vi "LoopVI-V3.vi"() -> ()   [LabVIEW 2013]
uses:
  <vilib>/Utility/file.llb/Read From Spreadsheet File (DBL).vi
panel:
  out "x*y":dbl
  out "Numeric":dbl format="%#_2f"
  in  "file path (dialog if empty)":path
  in  "Load":bool caption="measurement file\n\n         ??. txt"
  out "free gas model":cluster{"Y":dbl[], "Y":dbl[]}[](graph)
  in  "Fermi angle\n   (mrad)":dbl=7.0
  in  "stop 2":bool
  out "core electrons":cluster{"Y":dbl[], "Y":dbl[]}[](graph)
  in  "core width\n   (mrad)":dbl=5.0
  in  "fraction core\nannihilations":dbl=0.2 min=0.0 max=1.0 step=1e-05
  out "ZICHT  functie":cluster{"Y":dbl[], "Y":dbl[]}[](graph)
  in  "spleetbreedte\n      (mm)":dbl=1.0 min=0.1 max=5.0
  in  "collimator afstand\n       (mm)":dbl=500.0 min=100.0 max=1000.0
  in  "stop 4":bool
  out "XY Graph 4":cluster{ext[], "Array out":ext[]}[](graph)
  in  "alignment correction":dbl min=-10.0 max=10.0 step=0.0001
  in  "background \n coincidence counts":dbl min=0.0 max=100.0
  out "Fermi energy (eV)":dbl format="%#_3g"
  in  "22Na source radius (mm)":dbl=0.1 min=1e-05 max=3.0
  out "?":dbl format="%#_3g"
  in  "1d - Acar":bool caption="2d - Acar or DB"
  out "2d - Acar 2":bool
  out "2d - Acar 3":bool
  out "2d - Acar 4":bool
  out "XY Graph 5":cluster{ext[], "Array out":ext[]}[](graph)
  out "output cluster 2":cluster{ext[], ext[]}
  out "Sum of squared residuals":dbl
  in  "sigma (mrad) 2":dbl
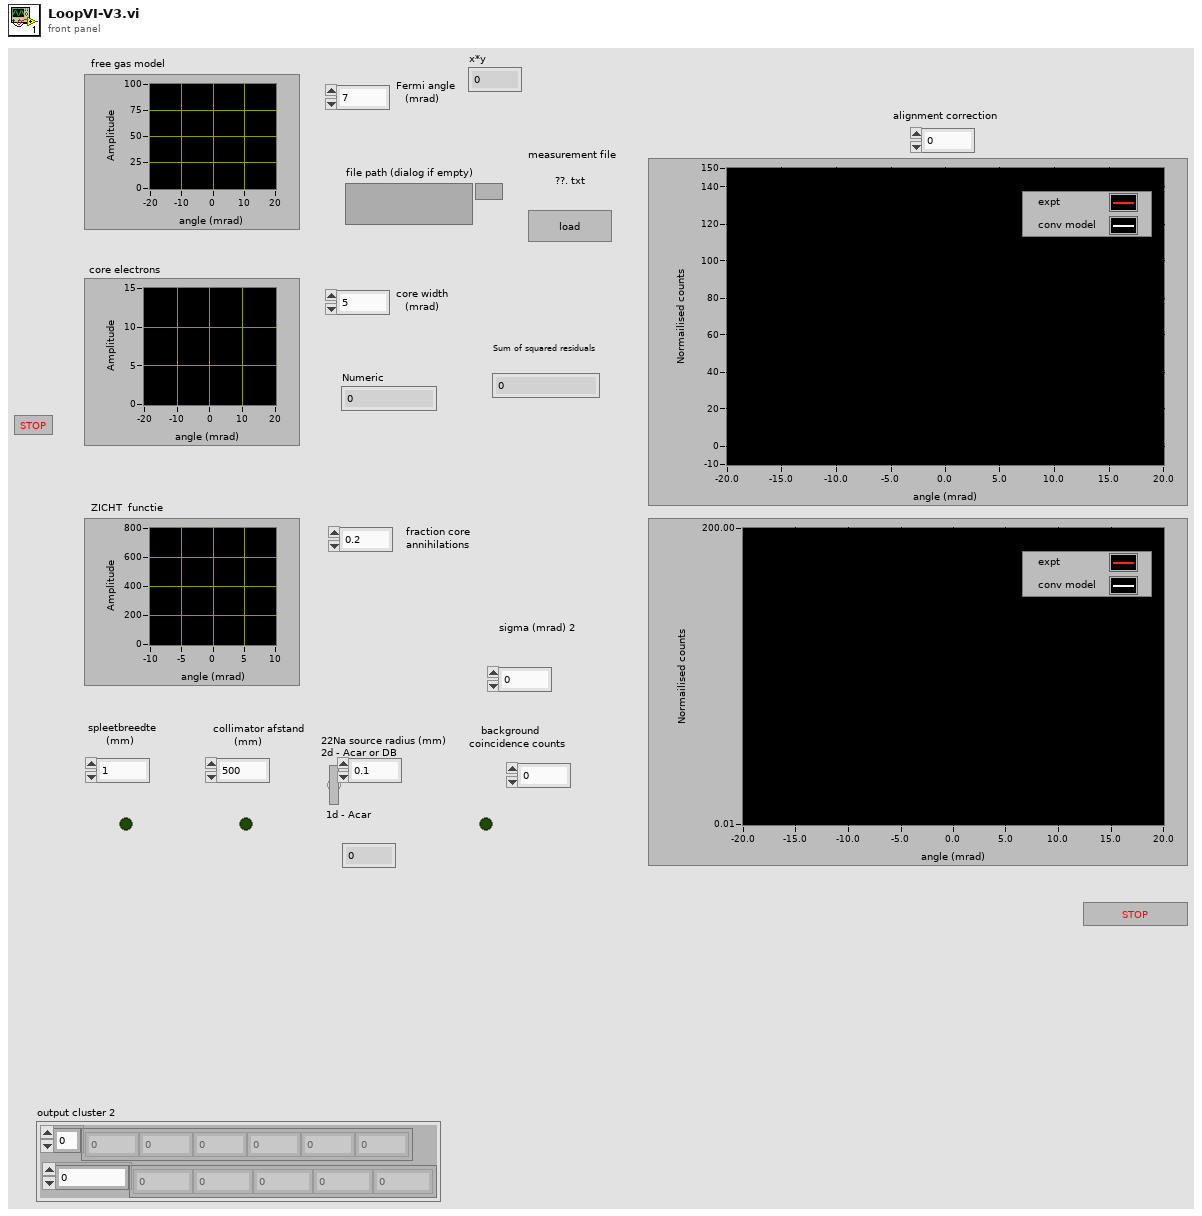
[diagram p1: front panel]
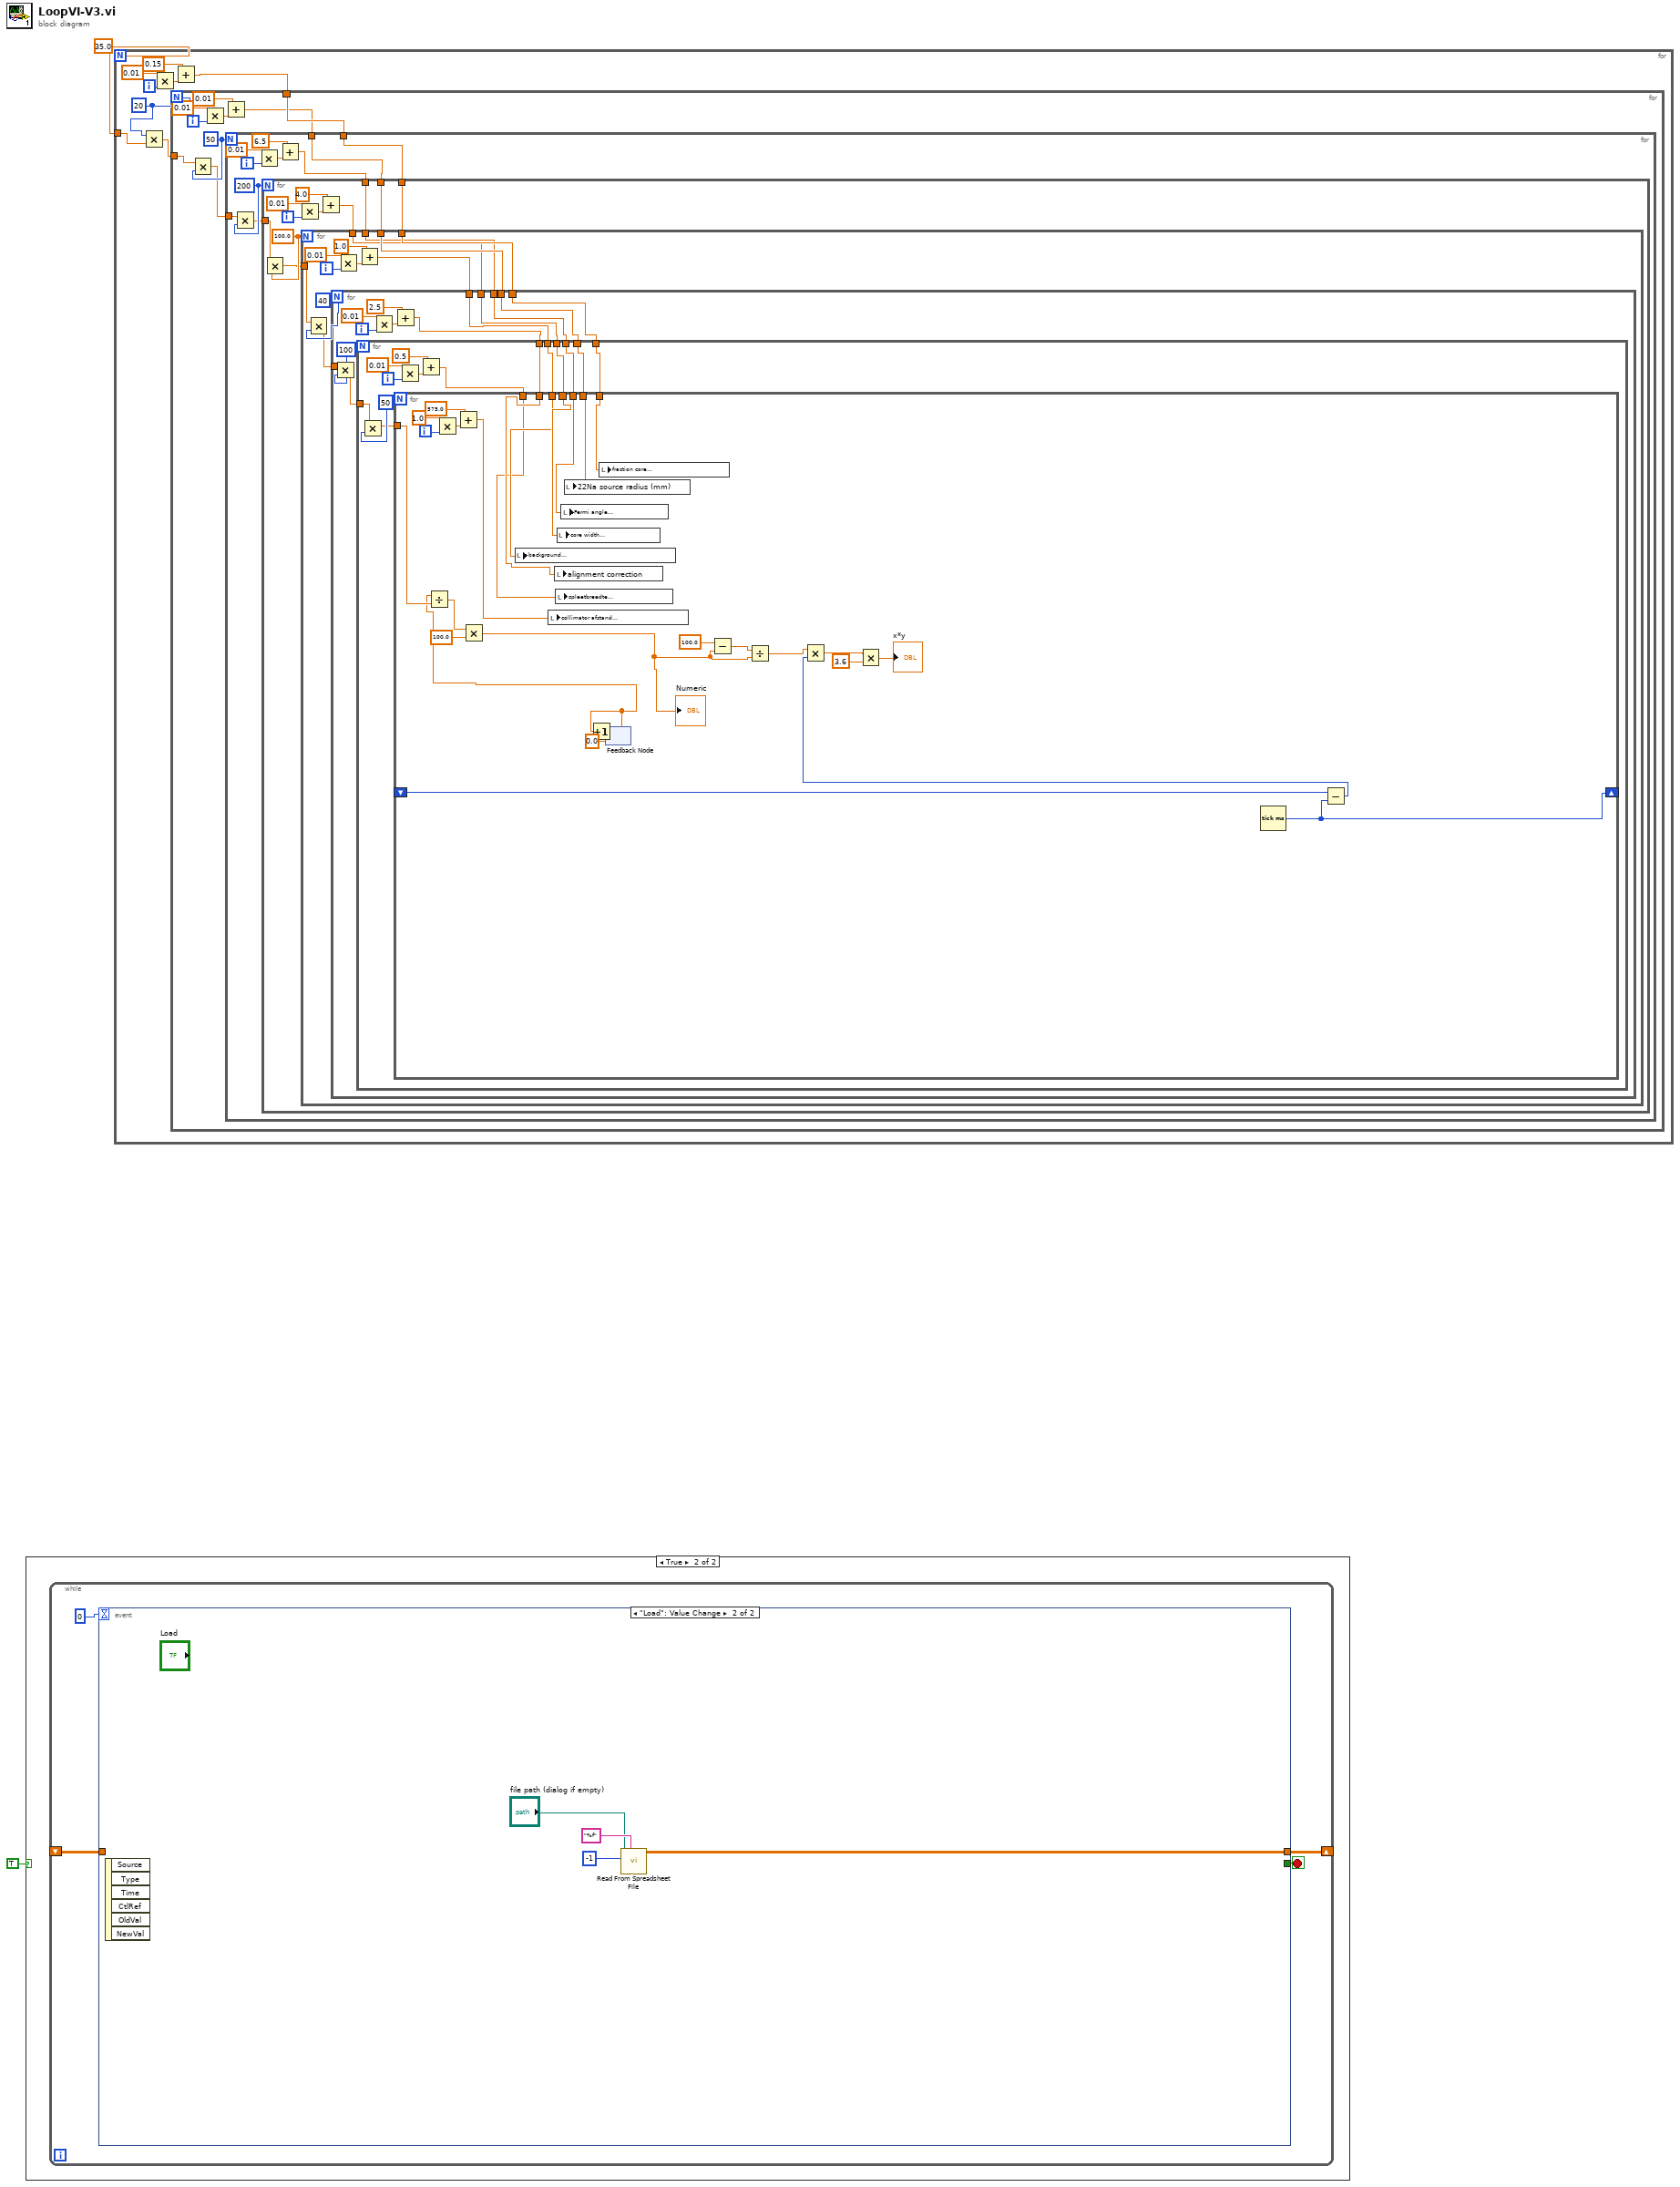
[diagram p0: block diagram]
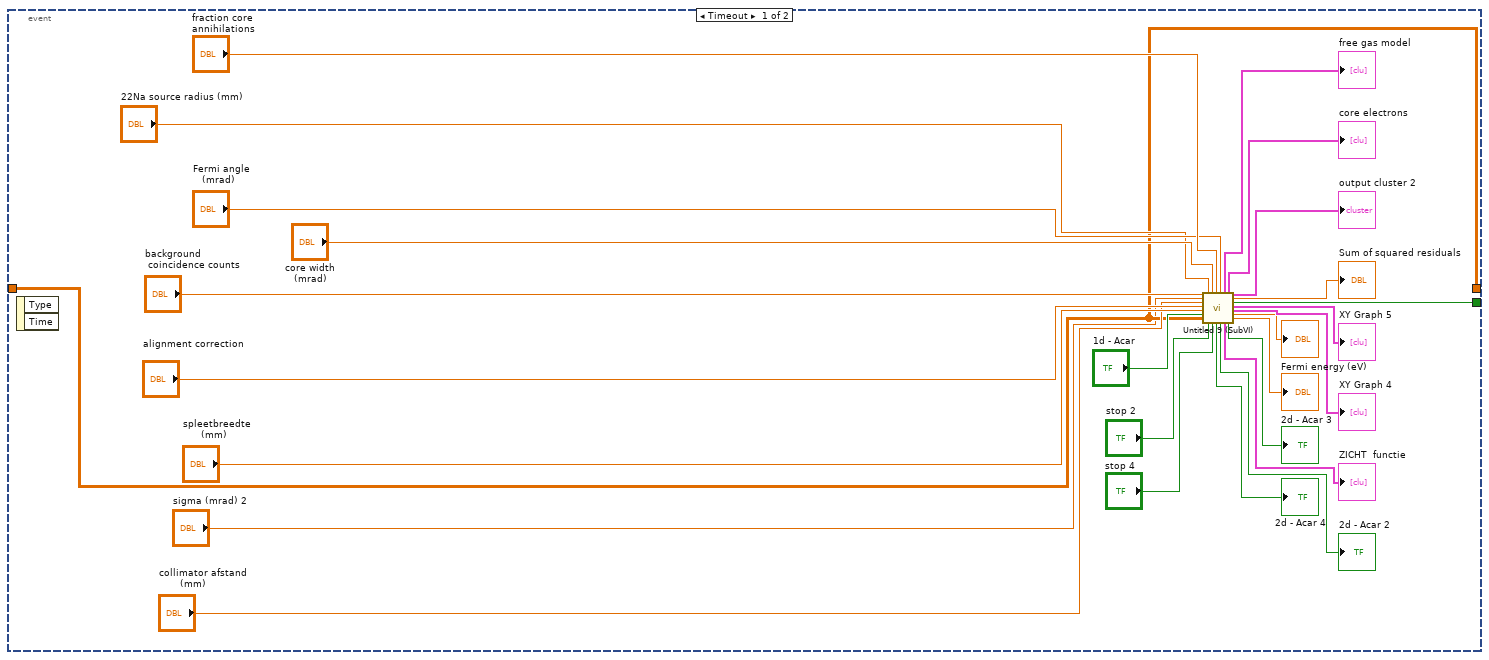
[diagram p3: hidden frame]
diagram:
  w1 = 35.0
  n1 = case shown="True" TRUE {
    frame False {
    }
    frame True {
      n2 = while {
        shift-right: [w4] -> _
        shift-left: _ -> [w3]
        stop <- w6 stop-if-true
        n3 = event shown="[1] \"Load\": Value Change" {
          selector: _ -> [_ _]
          dyn-events: _ -> [_ _]
          timeout: 0 -> [_ _]
          tunnel: [w32 _] -> w6
          tunnel: [w22 w35] -> w4
          tunnel: w3 -> [w22 _]
          event Timeout {
            n4 = event-data() -> ()  [unwired: 1 in, 2 out]
            n5 = call "Untitled 9 (SubVI).vi"("background \n coincidence counts"="background \n coincidence counts", "sigma (mrad) in"="sigma (mrad) 2", "collimator afstand\n       (mm)"="collimator afstand\n       (mm)", "alignment correction"="alignment correction", "spleetbreedte\n      (mm)"="spleetbreedte\n      (mm)", "1d - Acar"="1d - Acar", "all rows"=w22, "22Na source radius (mm)"="22Na source radius (mm)", "stop in"="stop 2", "core width\n   (mrad)"="core width\n   (mrad)", "stop 4"="stop 4", "fraction core\nannihilations"="fraction core\nannihilations", "Fermi angle\n   (mrad)"="Fermi angle\n   (mrad)") -> ("2d - Acar 4"=→"2d - Acar 4":bool, "2d - Acar 2"=→"2d - Acar 2":bool, "free gas model"=→"free gas model":cluster{"Y":dbl[], "Y":dbl[]}[], "ZICHT  functie"=→"ZICHT  functie":cluster{"Y":dbl[], "Y":dbl[]}[], "core electrons"=→"core electrons":cluster{"Y":dbl[], "Y":dbl[]}[], "2d - Acar 3"=→"2d - Acar 3":bool, "output cluster 2"=→"output cluster 2":cluster{ext[], ext[]}, "Sum of squared residuals"=→"Sum of squared residuals":dbl, "stop 3"=w32:bool, "XY Graph 5"=→"XY Graph 5":cluster{ext[], "Array out":ext[]}[], "XY Graph 4"=→"XY Graph 4":cluster{ext[], "Array out":ext[]}[], 25:→"?":dbl, "Fermi energy (eV)"=→"Fermi energy (eV)":dbl)  [unwired: 2 in]
          }
          event "Load": Value Change {
            n6 = event-data() -> ()  [unwired: 1 in, 6 out]
            n7 = call-poly <vilib>:"Read From Spreadsheet File.vi"("format (%.3f)"="%f", "number of rows (all:-1)"=-1, "file path (dialog if empty)"="file path (dialog if empty)") -> ("all rows"=w35:dbl[][])  [unwired: 4 in, 4 out]
          }
        }
      }
    }
  }
  n8 = for {
    N: w1 -> [_]
    tunnel: w1 -> [w39]
    i -> [w37]
    w40 = 20
    n9 = Multiply(x=w40, y=w39) -> (x*y=w38:dbl)
    n10 = Multiply(x=0.01, y=w37) -> (x*y=w43:dbl)
    n11 = Add(x=0.15, y=w43) -> (x+y=w41:dbl)
    n12 = for {
      N: w40 -> [_]
      tunnel: w41 -> [w49]
      tunnel: w38 -> [w47]
      i -> [w53]
      w46 = 50
      n13 = Multiply(x=w47, y=w46) -> (x*y=w45:dbl)
      n14 = Multiply(x=0.01, y=w53) -> (x*y=w51:dbl)
      n15 = Add(x=0.01, y=w51) -> (x+y=w48:dbl)
      n16 = for {
        N: w46 -> [_]
        tunnel: w49 -> [w59]
        tunnel: w48 -> [w58]
        tunnel: w45 -> [w56]
        i -> [w63]
        w55 = 200
        n17 = Multiply(x=w56, y=w55) -> (x*y=w54:dbl)
        n18 = Multiply(x=0.01, y=w63) -> (x*y=w61:dbl)
        n19 = Add(x=6.5, y=w61) -> (x+y=w57:dbl)
        n20 = for {
          N: w55 -> [_]
          tunnel: w59 -> [w67]
          tunnel: w58 -> [w68]
          tunnel: w57 -> [w69]
          tunnel: w54 -> [w66]
          i -> [w74]
          w65 = 100.0
          n21 = Multiply(x=w66, y=w65) -> (x*y=w64:dbl)
          n22 = Multiply(x=0.01, y=w74) -> (x*y=w72:dbl)
          n23 = Add(x=4.0, y=w72) -> (x+y=w70:dbl)
          n24 = for {
            N: w65 -> [_]
            tunnel: w70 -> [w79]
            tunnel: w69 -> [w80]
            tunnel: w68 -> [w81]
            tunnel: w67 -> [w82]
            tunnel: w64 -> [w77]
            i -> [w86]
            w76 = 40
            n25 = Multiply(x=w77, y=w76) -> (x*y=w75:dbl)
            n26 = Multiply(x=0.01, y=w86) -> (x*y=w84:dbl)
            n27 = Add(x=1.0, y=w84) -> (x+y=w78:dbl)
            n28 = for {
              N: w76 -> [_]
              tunnel: w82 -> [w95]
              tunnel: w81 -> [w94]
              tunnel: w80 -> [w93]
              tunnel: w79 -> [w92]
              tunnel: w78 -> [w91]
              tunnel: w75 -> [w89]
              i -> [w99]
              w88 = 100
              n29 = Multiply(x=w89, y=w88) -> (x*y=w87:dbl)
              n30 = Multiply(x=0.01, y=w99) -> (x*y=w97:dbl)
              n31 = Add(x=2.5, y=w97) -> (x+y=w90:dbl)
              n32 = for {
                N: w88 -> [_]
                tunnel: w95 -> [w108]
                tunnel: w94 -> [w107]
                tunnel: w93 -> [w106]
                tunnel: w92 -> [w105]
                tunnel: w91 -> [w104]
                tunnel: w90 -> [w103]
                tunnel: w87 -> [w102]
                i -> [w113]
                w101 = 50
                n33 = Multiply(x=w102, y=w101) -> (x*y=w100:dbl)
                n34 = Multiply(x=0.01, y=w113) -> (x*y=w111:dbl)
                n35 = Add(x=0.5, y=w111) -> (x+y=w109:dbl)
                n36 = for {
                  N: w101 -> [_]
                  tunnel: w109 -> [w131]
                  tunnel: w108 -> [w137]
                  tunnel: w107 -> [w136]
                  tunnel: w106 -> [w135]
                  tunnel: w105 -> [w134]
                  tunnel: w104 -> [w133]
                  tunnel: w103 -> [w132]
                  tunnel: w100 -> [w127]
                  shift-right: [w119] -> _
                  shift-left: _ -> [w123]
                  i -> [w141]
                  n37 = Multiply(x=1.0, y=w141) -> (x*y=w139:dbl)
                  n38 = Add(x=575.0, y=w139) -> (x+y=w130:dbl)
                  n39 = local write "background \n coincidence counts"(w133) -> ()
                  n40 = local write "collimator afstand\n       (mm)"(w130) -> ()
                  n41 = local write "alignment correction"(w132) -> ()
                  n42 = local write "spleetbreedte\n      (mm)"(w131) -> ()
                  n43 = local write "core width\n   (mrad)"(w134) -> ()
                  n44 = local write "Fermi angle\n   (mrad)"(w135) -> ()
                  n45 = local write "22Na source radius (mm)"(w136) -> ()
                  n46 = local write "fraction core\nannihilations"(w137) -> ()
                  n47 = feedback #1(0.0) -> (w126:dbl)
                  n48 = Divide(x=w126, y=w127) -> (x/y=w125:dbl)
                  n49 = Multiply(x=w125, y=100.0) -> (x*y=w120:dbl)
                  "Numeric" <- w120
                  n50 = Increment(x=w126) -> (x+1=w129:dbl)
                  n51 = feedback-in #1(w129) -> ()
                  n52 = Subtract(x=100.0, y=w120) -> (x-y=w121:dbl)
                  n53 = Divide(x=w121, y=w120) -> (x/y=w118:dbl)
                  n54 = Tick Count (ms)() -> (millisecond timer value=w119:u32)
                  n55 = Subtract(x=w123, y=w119) -> (x-y=w117:u32)
                  n56 = Multiply(x=w118, y=w117) -> (x*y=w116:dbl)
                  n57 = Multiply(x=w116, y=3.6) -> (x*y=→"x*y":dbl)
                }
              }
            }
          }
        }
      }
    }
  }
